vi "BalanceMotorControl2.vi"(8 "Number of Motors":i16) -> ()   [LabVIEW 2019]
panel:
  out "error out 2":errorcluster
  in  "Boolean":bool
  out "error out":errorcluster
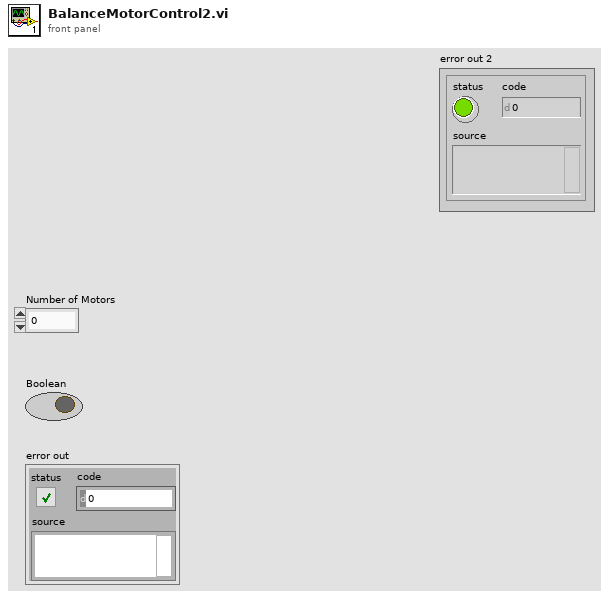
[diagram p1: front panel]
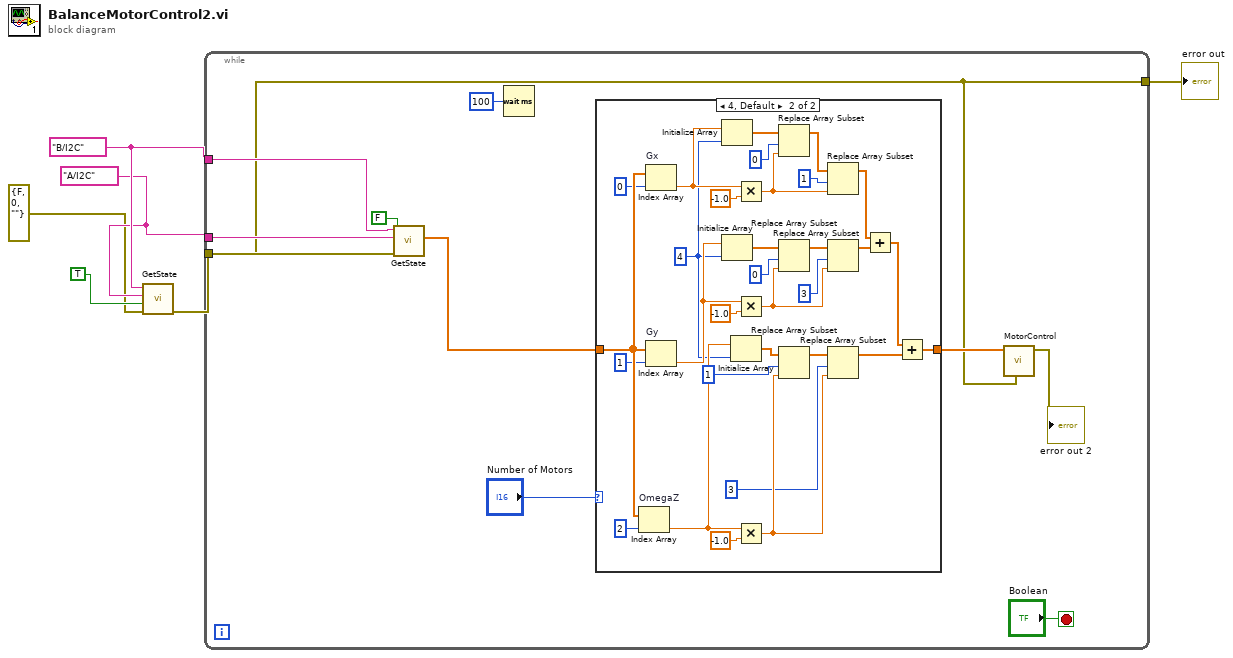
[diagram p0: block diagram]
diagram:
  w3 = tag "A/I2C" ("IMU Channel")
  w5 = tag "B/I2C" ("LIDAR Channel")
  n1 = call "GetState.vi"("error in (no error)"=errorcluster {"status"=FALSE, "code"=0, "source"=""}, "Calibrate?"=TRUE, "IMU Channel"=w3, "LIDAR Channel"=w5) -> ("error out"=w4:errorcluster)  [unwired: 2 in, 3 out]
  n2 = while {
    tunnel: w5 -> [w14]
    tunnel: w4 -> [w13]
    tunnel: w3 -> [w12]
    tunnel: [w9] -> w2
    stop <- "Boolean" stop-if-true
    n3 = call "GetState.vi"("error in (no error)"=w13, "Calibrate?"=FALSE, "IMU Channel"=w12, "LIDAR Channel"=w14) -> ("error out"=w9:errorcluster, "Angular Velocity"=w8:dbl[])  [unwired: 2 in, 2 out]
    n4 = Wait (ms)(milliseconds to wait=u32 100) -> ()  [unwired: 1 out]
    n5 = case shown="4, Default" "Number of Motors" {
      tunnel: w8 -> [w18 w49]
      tunnel: [w18 w29] -> w16
      frame 6 {
      }
      frame 4, Default {
        w22 = 4 ("dimension size")
        n6 = Index Array "OmegaZ"(array=w49, index=2) -> (element=w45:dbl)
        n7 = Index Array "Gx"(array=w49, index=0) -> (element=w48:dbl)
        n8 = Index Array "Gy"(array=w49, index=1) -> (element=w46:dbl)
        n9 = Initialize Array(w48, w22) -> (w42:dbl[])
        n10 = Initialize Array(w46, w22) -> (w39:dbl[])
        n11 = Initialize Array(w45, w22) -> (w36:dbl[])
        n12 = Multiply(x=w48, y=-1.0) -> (x*y=w40:dbl)
        n13 = Multiply(x=w46, y=-1.0) -> (x*y=w37:dbl)
        n14 = Multiply(x=w45, y=-1.0) -> (x*y=w34:dbl)
        n15 = Replace Array Subset(array=w42, new element=w40, index=0) -> (w41:dbl[])
        n16 = Replace Array Subset(array=w39, new element=w37, index=0) -> (w38:dbl[])
        n17 = Replace Array Subset(array=w36, new element=w34, index=i16 1 ("Motors 1 or 3")) -> (w35:dbl[])
        n18 = Replace Array Subset(array=w41, new element=w40, index=1) -> (w33:dbl[])
        n19 = Replace Array Subset(array=w38, new element=w37, index=3) -> (w32:dbl[])
        n20 = Replace Array Subset(array=w35, new element=w34, index=i16 3 ("Motors 2 or 4")) -> (w31:dbl[])
        n21 = Add(x=w33, y=w32) -> (x+y=w30:dbl[])
        n22 = Add(x=w30, y=w31) -> (x+y=w29:dbl[])
      }
    }
    n23 = call "MotorControl.vi"("error in (no error)"=w9, "Array"=w16) -> ("error out"=→"error out 2":errorcluster)  [unwired: 9 in]
  }
  "error out" <- w2
